vi "Delete Directory.vi"(8 "Error In":errorcluster, 10 "Remote Path":string, 11 "SFTP In":refnum<class "SFTP.lvclass">) -> (0 "Error Out":errorcluster, 3 "SFTP Out":refnum<class "SFTP.lvclass">)   [LabVIEW 2018, in "Toolkit.lvlib" / "SFTP.lvclass"]
doc: "Destroys, a.k.a. deletes or removes, a directory from the remote SFTP server."
uses:
  SFTP.lvclass
  SFTP.lvclass/SFTP.ctl
  Session/Session.lvclass/Session.ctl
  SSH/SSH.lvclass/SSH.ctl
  Toolkit.lvlib
  Session/Session.lvclass
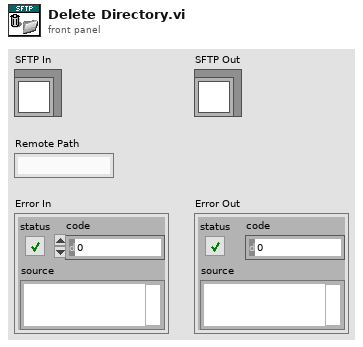
[diagram p1: front panel]
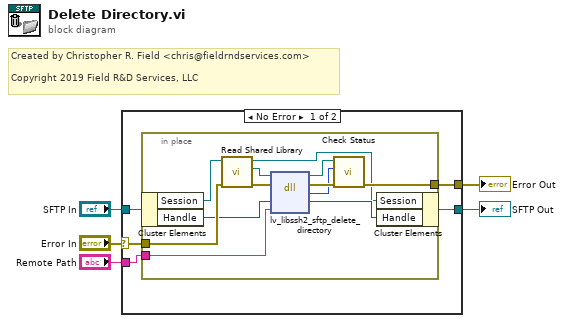
[diagram p0: block diagram]
diagram:
  # "Created by Christopher R. Field <chris@fieldrndservices.com>\n\nCopyright 2019 Field R&D Services, LLC"
  n1 = case shown="No Error" "Error In" {
    selector: "Error In" -> [w10 w24]
    tunnel: [w9 w24] -> w4
    tunnel: "SFTP In" -> [w8 w23]
    tunnel: [w7 w23] -> w2
    tunnel: "Remote Path" -> [w6 _]
    frame No Error {
      n2 = in-place {
        in-place-border: w10 -> [w17]
        in-place-border: [w18] -> w9
        in-place-border: w6 -> [w11]
        n3 = in-place-cluster #1(w8) -> ("Session"=w16:refnum<class "Session.lvclass">, "Handle"=w12:u64)
        n4 = call "Read Shared Library.vi"("Error In"=w17, "Session In"=w16) -> ("Erorr Out"=w14:errorcluster, "libssh2lv Shared Library"=w13:path, "Session Out"=w15:refnum<class "Session.lvclass">)  [unwired: 7 in]
        n5 = dll-call lib="libssh2lv.*" fn="lv_libssh2_sftp_delete_directory"(path in=w13, error in=w14, "handle"=w12, "directory_path"=w11) -> (path out=w20:path, error out=w21:errorcluster, "status"=w19:i32, "handle"=w22:u64)  [unwired: 2 in]
        n6 = call "Check Status.vi"("Error In"=w21, "Status"=w19, "libssh2lv Shared Library In"=w20) -> ("Error Out"=w18:errorcluster)  [unwired: 7 in, 1 out]
        n7 = in-place-cluster #1("Session"=w15, "Handle"=w22) -> (w7:refnum<class "SFTP.lvclass">)
      }
    }
    frame Error {
    }
  }
  "Error Out" <- w4
  "SFTP Out" <- w2
